vi "Initialize.vi"(8 "error in (no error)":errorcluster, 9 "Components":refnum<class "Component.lvclass">[](array[class]), 10 "group configuration":T3, 11 "Group Configuration in":refnum<class "Group Configuration.lvclass">) -> (0 "error out":errorcluster, 3 "Group Configuration out":refnum<class "Group Configuration.lvclass">)   [LabVIEW 2017, in "DSF Core.lvlib" / "Group Configuration.lvclass"]
uses:
  Group Configuration.lvclass
  Component/Component.lvclass
  Typedefs/DSF Component Configuration.ctl
  Typedefs/DSF Version Info.ctl
  DSF Core.lvlib
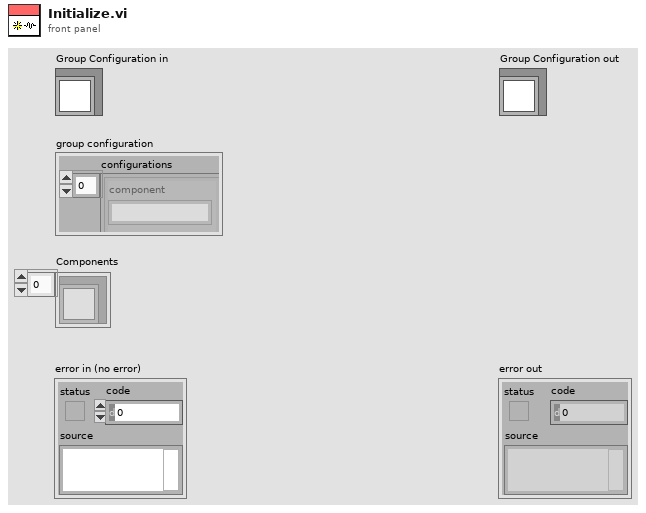
[diagram p1: front panel]
types:
  T1 = typedef "DSF Core.lvlib/DSF Component Configuration.ctl" = cluster{"component":string, "data":string, "data version":T2}
  T2 = typedef "DSF Core.lvlib/DSF Version Info.ctl" = cluster{"major":i32, "minor":i32, "fix":i32, "build":string}
  T3 = cluster{"configurations":T1[], "transfers":cluster{"configurations":T1[]}[]}
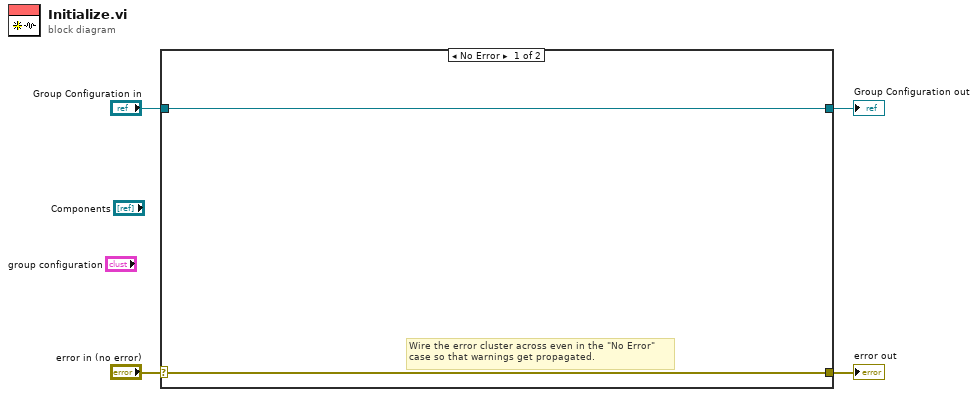
[diagram p0: block diagram]
diagram:
  n1 = case shown="No Error" "error in (no error)" {
    selector: "error in (no error)" -> [w5 w8]
    tunnel: [w5 w8] -> w3
    tunnel: [w6 w7] -> w1
    tunnel: "Group Configuration in" -> [w6 w7]
    frame No Error {
      # "Wire the error cluster across even in the \"No Error\"\ncase so that warnings get propagated."
    }
    frame Error {
    }
  }
  "error out" <- w3
  "Group Configuration out" <- w1
